vi "basic baza.vi"   [LabVIEW 2023]
uses:
  <vilib>/Utility/file.llb/Write Delimited Spreadsheet (string).vi
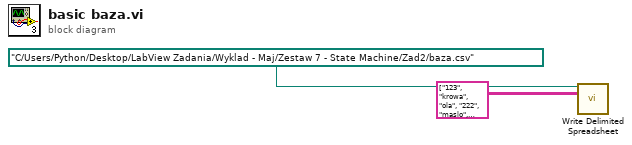
[diagram p0: block diagram]
diagram:
  n1 = call-poly <vilib>:"Write Delimited Spreadsheet.vi"("file path (dialog if empty)"=path "C:/Users/Python/Desktop/LabView Zadania/Wyklad - Maj/Zestaw 7 - State Machine/Zad2/baza.csv", "2D data"=string[][] [["123", "krowa", "ola"], ["222", "maslo", "mateusz"], ["33", "kurczak", "michal"], ["443", "myszka", "jan"], ["22", "laptop", "andrzej"], ["1", "olowek", "krzysztof"], ["4", "dlugopis", "agnieszka"], ["2", "zeszyt", "tomek"], ["3", "drewno", "marcel"]] ("Dane")) -> ()  [unwired: 12 in, 2 out]
